vi "_RT_CtrlLoop_D999_Read_VISA.vi"(8 "error in (no error)":errorcluster, 10 "Comm Str":string, 11 "VISA resource In":refnum<visa-resource-name>) -> (0 "error out":errorcluster, 1 "Is Exist?":bool, 2 "Response Str":string, 3 "VISA resource Out":refnum<visa-resource-name>)   [LabVIEW 2018]
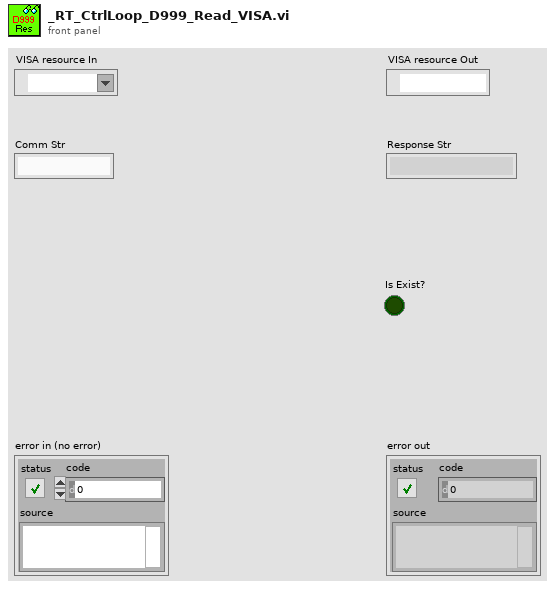
[diagram p1: front panel]
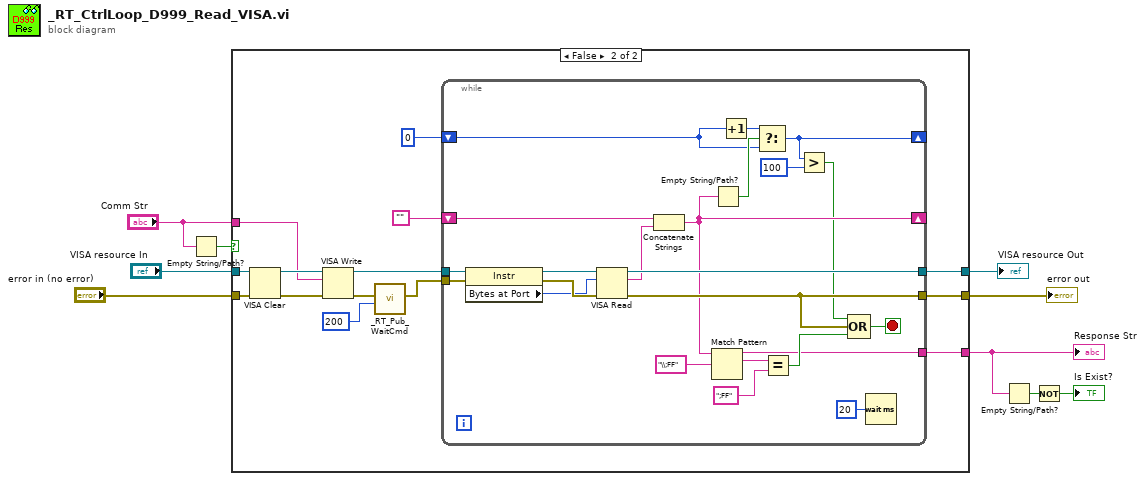
[diagram p0: block diagram]
diagram:
  n1 = Empty String/Path?(string/path="Comm Str") -> (empty?=w2:bool)
  n2 = case shown="False" w2 {
    tunnel: [_ w18] -> w7
    tunnel: "VISA resource In" -> [w11 w17]
    tunnel: "error in (no error)" -> [w10 w16]
    tunnel: [w10 w15] -> w4
    tunnel: [w11 w14] -> w3
    tunnel: "Comm Str" -> [_ w13]
    frame True {
    }
    frame False {
      n3 = VISA Clear(VISA resource name=w17, error in (no error)=w16) -> (VISA resource name out=w25:refnum<visa-resource-name>, error out=w24:errorcluster)
      n4 = VISA Write(VISA resource name=w25, write buffer=w13, error in (no error)=w24) -> (VISA resource name out=w23:refnum<visa-resource-name>, error out=w22:errorcluster)  [unwired: 1 out]
      n5 = call "_RT_Pub_WaitCmd.vi"("milliseconds to wait"=u32 200, "error in (no error)"=w22) -> ("error out"=w21:errorcluster)  [unwired: 9 in]
      n6 = while {
        shift-right: [w27] -> _
        shift-left: "" -> [w33]
        tunnel: [w48] -> w14
        tunnel: [w44] -> w15
        tunnel: w23 -> [w39]
        tunnel: w21 -> [w38]
        tunnel: [w34] -> w18
        shift-right: [w29] -> _
        shift-left: 0 -> [w30]
        stop <- w42 stop-if-true
        n7 = property class="Instr"(reference=w39, error in=w38) -> (reference out=w40:refnum<visa-resource-name>, error out=w41:errorcluster, "Bytes at Port"=w37:u32)
        n8 = VISA Read(VISA resource name=w40, byte count=w37, error in (no error)=w41) -> (VISA resource name out=w48:refnum<visa-resource-name>, read buffer=w35:string, error out=w44:errorcluster)  [unwired: 1 out]
        n9 = Concatenate Strings(w33, w35) -> (w27:string)
        n10 = Match Pattern(string=w27, regular expression="\\;FF") -> (before substring=w34:string, match substring=w46:string)  [unwired: 1 in, 2 out]
        n11 = Empty String/Path?(string/path=w27) -> (empty?=w32:bool)
        n12 = Increment(x=w30) -> (x+1=w31:i32)
        n13 = Select(t=w31, s=w32, f=w30) -> (s? t:f=w29:i32)
        n14 = Equal?(x=w46, y=";FF") -> (x = y?=w43:bool)
        n15 = Greater?(x=w29, y=100) -> (0:w26:bool)
        n16 = Compound Arithmetic op=OR(w26, w44, w43) -> (w42:bool)
        n17 = Wait (ms)(milliseconds to wait=u32 20) -> ()  [unwired: 1 out]
      }
    }
  }
  "error out" <- w4
  "VISA resource Out" <- w3
  "Response Str" <- w7
  n18 = Empty String/Path?(string/path=w7) -> (empty?=w9:bool)
  n19 = Not(x=w9) -> (.not. x?=→"Is Exist?":bool)
